vi "global_variable.vi"() -> ()   [LabVIEW 2023]
panel:
  out "全局时间":string
  out "匹配行数":dbl
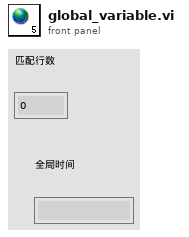
[diagram p1: front panel]
diagram:
